vi "Log.vi"(7 "Enum Coordenadas":T4, 8 "Error In":errorcluster, 9 "Confirmação":bool, 10 "Log States":T5, 11 "DataIn":T1={"Quem Joga"="", "Tabuleiro"={"(0,0)"="", "(1,0)"="", "(0,1)"="", "(1,1)"="", "(2,0)"="", "(1,2)"="", "(2,2)"="", "(0,2)"="", "(2,1) "=""}, "GameOption"=enum."Multiplayer local", "Turno"=FALSE, "Player"="", "Player 1"="", "Player 2"="", "Dificuldade"=enum."Easy", "Table"=[], "Row"=0, "Aceitar Convite"=FALSE, "Inviter line"=0, "diretório"=path "", "Logout - panel close"=FALSE, "StartGame"=FALSE, "MatchData.lvclass"=refnum, "GameMode"=enum."Single Easy", "Level State"=FALSE}) -> (0 "Error Out":errorcluster, 3 "DataIn 2":T1={"Quem Joga"="", "Tabuleiro"={"(0,0)"="", "(1,0)"="", "(0,1)"="", "(1,1)"="", "(2,0)"="", "(1,2)"="", "(2,2)"="", "(0,2)"="", "(2,1) "=""}, "GameOption"=enum."Multiplayer local", "Turno"=FALSE, "Player"="", "Player 1"="", "Player 2"="", "Dificuldade"=enum."Easy", "Table"=[], "Row"=0, "Aceitar Convite"=FALSE, "Inviter line"=0, "diretório"=path "", "Logout - panel close"=FALSE, "StartGame"=FALSE, "MatchData.lvclass"=refnum, "GameMode"=enum."Single Easy", "Level State"=FALSE})   [LabVIEW 2018]
doc: "SubVI criada para fazer o log do histórico de partida jogada a jogada, registrando o vencedor."
uses:
  controls/LogStates.ctl
  controls/TabuleiroCoordenadas.ctl
  controls/DataIn.ctl
  MatchDataClasses/MatchData/MatchData.lvclass
  controls/Tabuleiro.ctl
  controls/Table.ctl
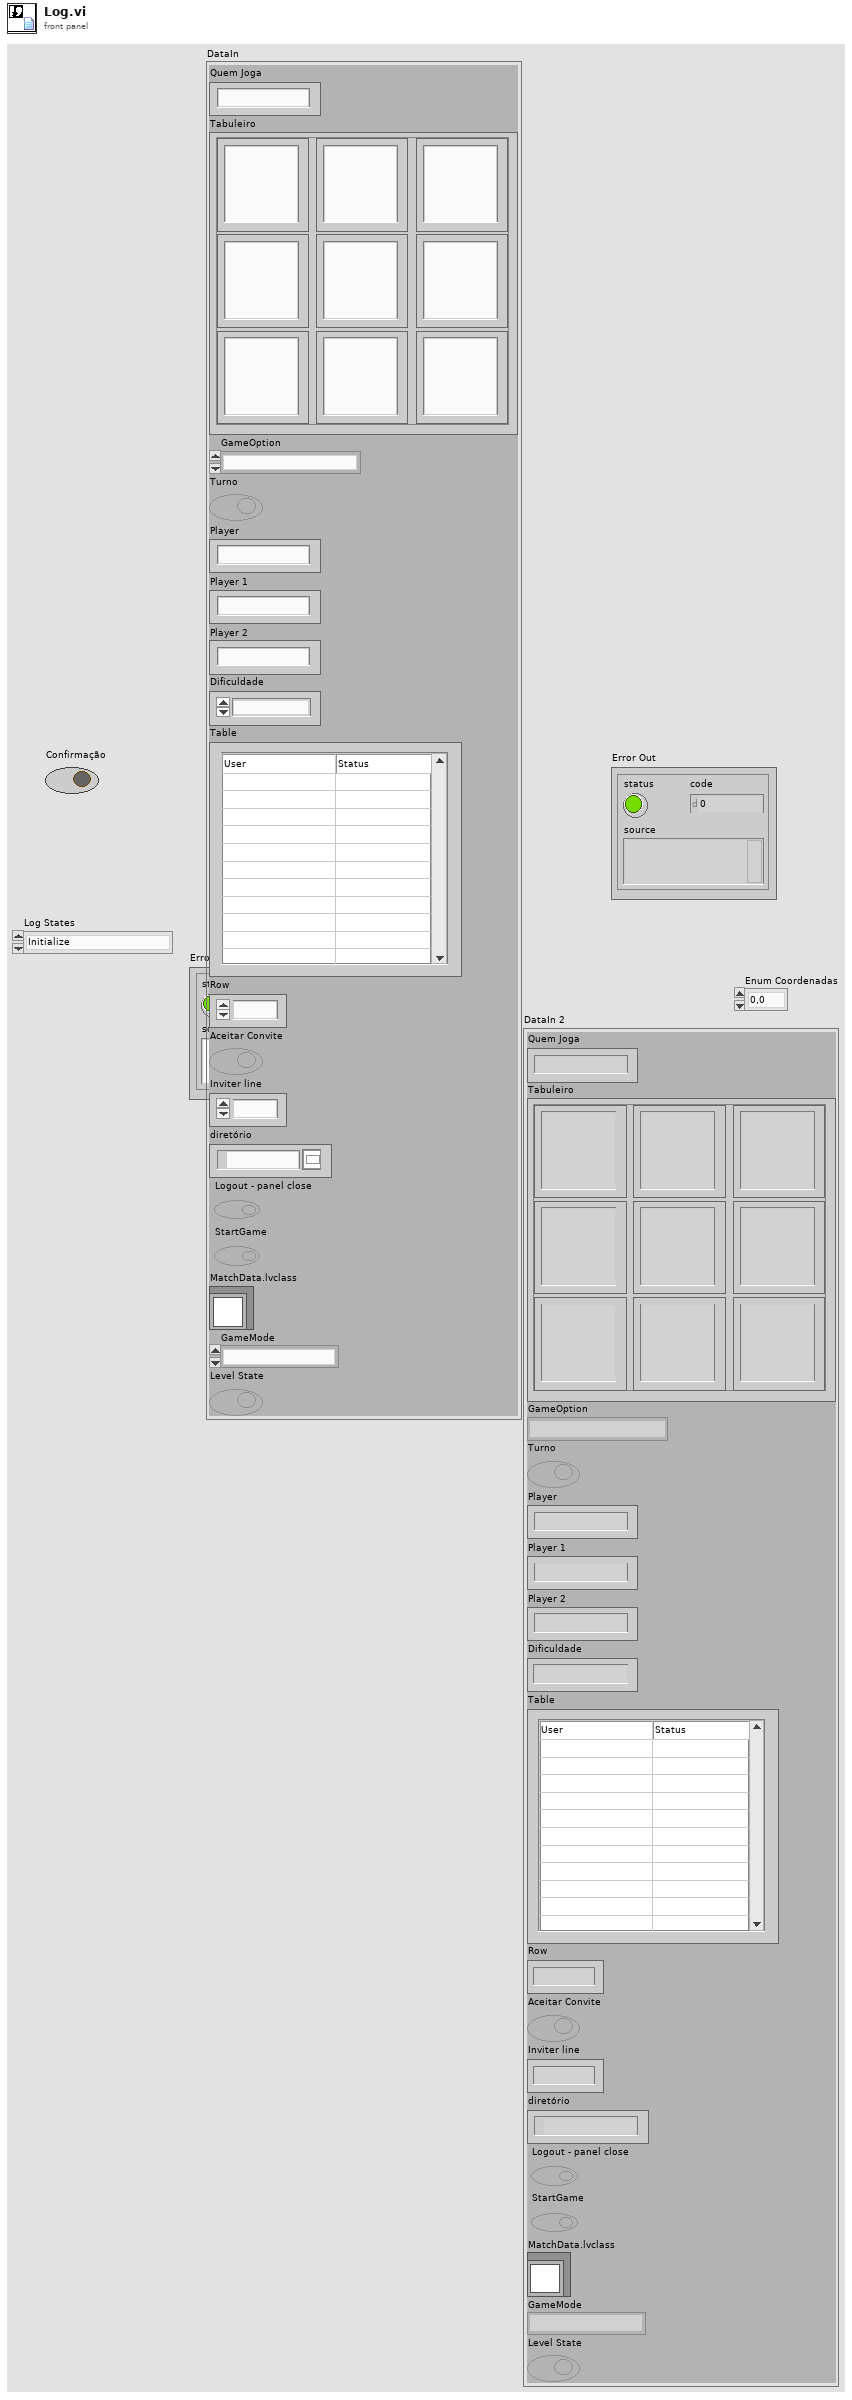
[diagram p1: front panel]
types:
  T1 = typedef "DataIn.ctl" = cluster{"Quem Joga":string, "Tabuleiro":T2, "GameOption":enum16{"Single Player", "Multiplayer local", "Multiplayer remoto", "Wait for Event", "Initialize", "Stop"}, "Turno":bool, "Player":string, "Player 1":string, "Player 2":string, "Dificuldade":enum16{"Easy", "Medium", "Hard"}, "Table":T3, "Row":u32, "Aceitar Convite":bool, "Inviter line":u32, "diretório":path, "Logout - panel close":bool, "StartGame":bool, "MatchData.lvclass":refnum<class "MatchData.lvclass">, "GameMode":enum16{"Single Easy", "Single Medium", "Single Hard", "Local", "Remote"}, "Level State":bool}
  T2 = typedef "Tabuleiro.ctl" = cluster{"(0,0)":string, "(1,0)":string, "(0,1)":string, "(1,1)":string, "(2,0)":string, "(1,2)":string, "(2,2)":string, "(0,2)":string, "(2,1) ":string}
  T3 = typedef "Table.ctl" = string[][]
  T4 = typedef "TabuleiroCoordenadas.ctl" = enum16{"0,0", "0,1", "0,2", "1,0", "1,1", "1,2", "2,0", "2,1", "2,2"}
  T5 = typedef "LogStates.ctl" = enum16{"Initialize", "Write", "Write (win, draw)", "Write (PC first)", "Write (Player first)", "Close"}
  T6 = enum16{"open", "replace", "create", "open or create", "replace or create", "replace or create with confirmation"}
  T7 = enum16{"Single Player", "Multiplayer local", "Multiplayer remoto", "Wait for Event", "Initialize", "Stop"}
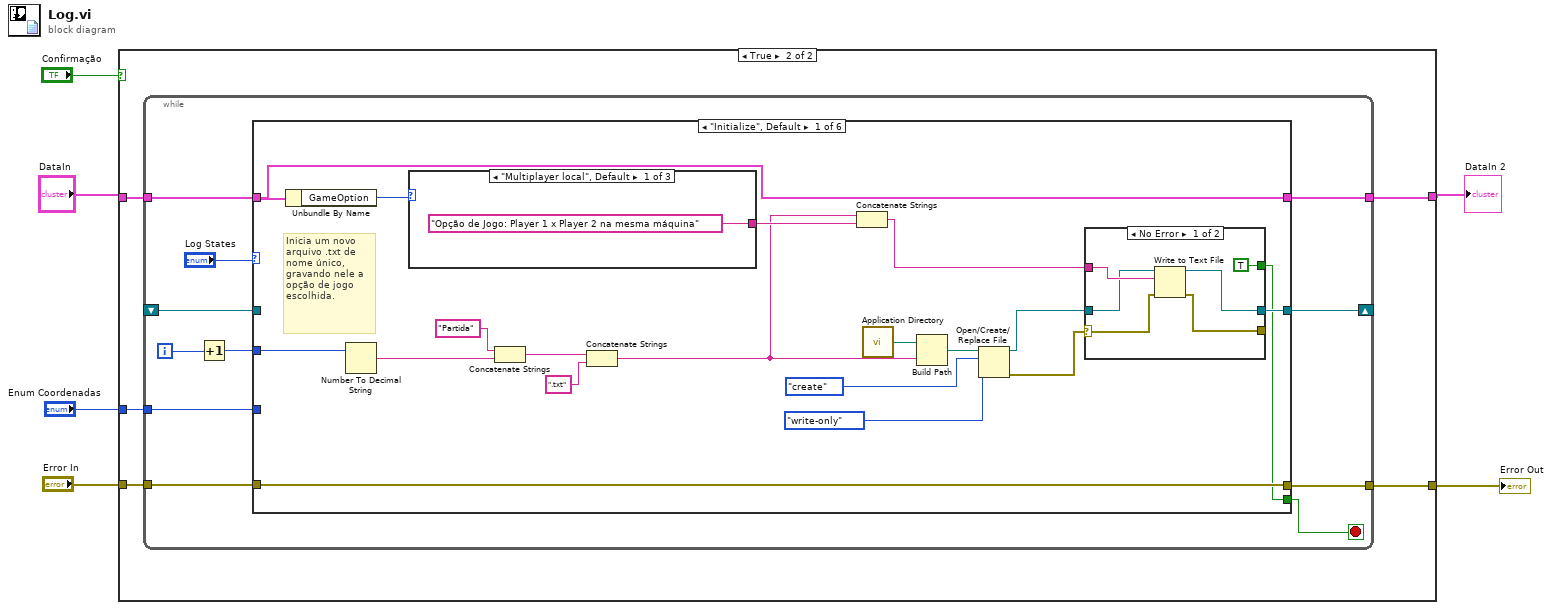
[diagram p0: block diagram]
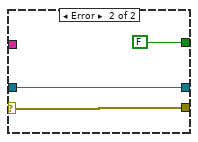
[diagram p3: hidden frame]
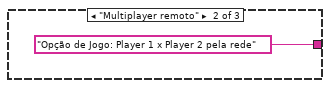
[diagram p4: hidden frame]
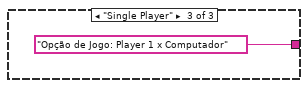
[diagram p5: hidden frame]
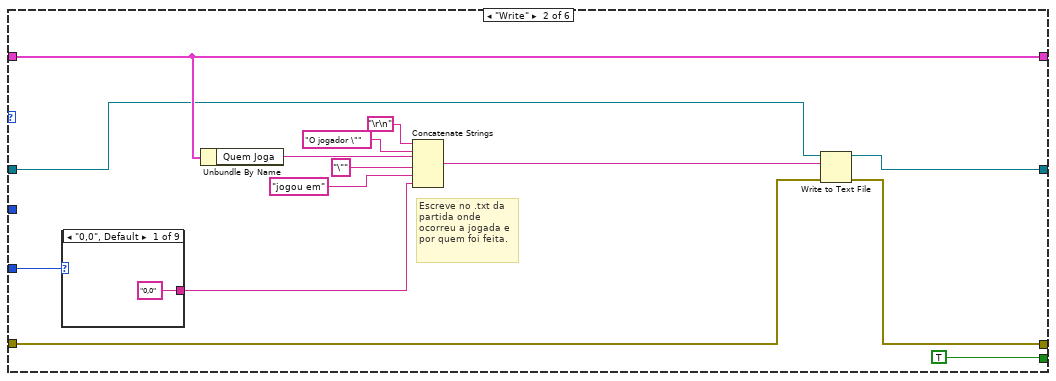
[diagram p6: hidden frame]
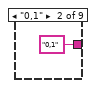
[diagram p7: hidden frame]
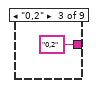
[diagram p8: hidden frame]
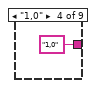
[diagram p9: hidden frame]
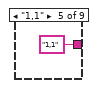
[diagram p10: hidden frame]
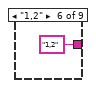
[diagram p11: hidden frame]
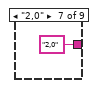
[diagram p12: hidden frame]
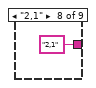
[diagram p13: hidden frame]
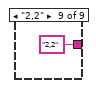
[diagram p14: hidden frame]
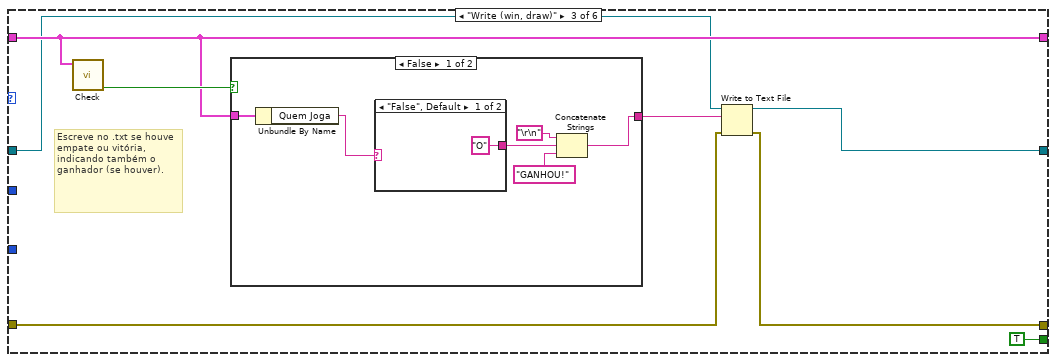
[diagram p15: hidden frame]
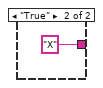
[diagram p16: hidden frame]
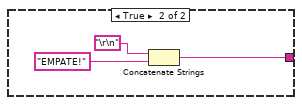
[diagram p17: hidden frame]
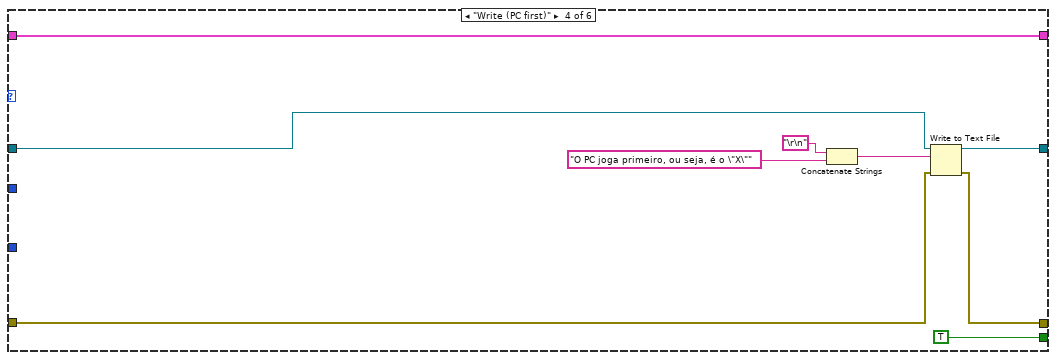
[diagram p18: hidden frame]
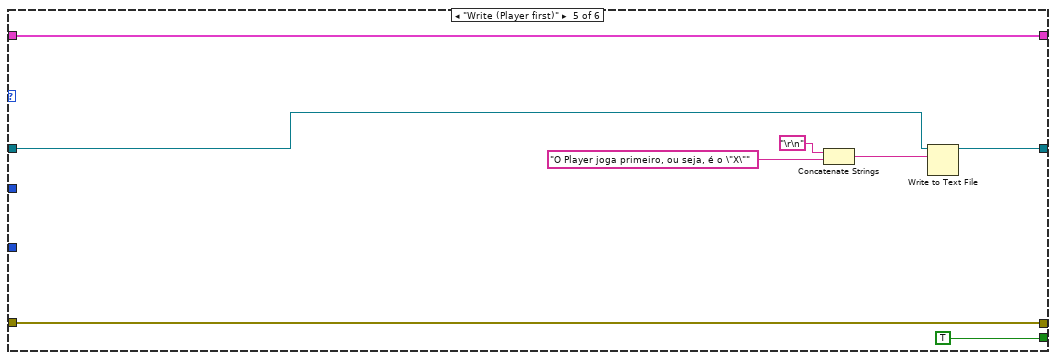
[diagram p19: hidden frame]
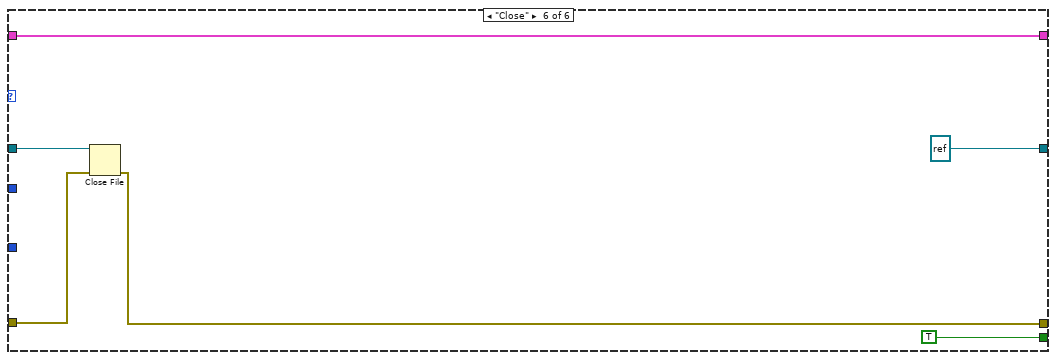
[diagram p20: hidden frame]
diagram:
  n1 = case shown="True" "Confirmação" {
    tunnel: "DataIn" -> [w8 w13]
    tunnel: "Error In" -> [w7 w12]
    tunnel: "Enum Coordenadas" -> [_ w11]
    tunnel: [w8 w10] -> w1
    tunnel: [w7 w9] -> w3
    frame False {
    }
    frame True {
      n2 = while {
        tunnel: w13 -> [w21]
        tunnel: w12 -> [w19]
        tunnel: w11 -> [w20]
        shift-right: [w18] -> _
        shift-left: _ -> [w17]
        tunnel: [w16] -> w10
        tunnel: [w15] -> w9
        i -> [w23]
        stop <- w14 stop-if-true
        n3 = Increment(x=w23) -> (x+1=w22:i32)
        n4 = case shown="\"Initialize\", Default" "Log States" {
          tunnel: w22 -> [w41 _ _ _ _ _]
          tunnel: w21 -> [w43 w65 w84 w106 w114 w117]
          tunnel: w20 -> [_ w68 _ _ _ _]
          tunnel: w19 -> [w26 w59 w82 w103 w113 w118]
          tunnel: [w27 w56 w80 w104 w108 refnum<file> refnum ("refnum out")] -> w18
          tunnel: w17 -> [_ w57 w79 w98 w107 w119]
          tunnel: [w43 w65 w84 w106 w114 w117] -> w16
          tunnel: [w26 w58 w81 w102 w113 w116] -> w15
          tunnel: [w25 TRUE TRUE TRUE TRUE TRUE] -> w14
          frame "Initialize", Default {
            # "Inicia um novo arquivo .txt de nome único, gravando nele a opção de jogo escolhida."
            n5 = Unbundle By Name(w43) -> ("GameOption"=w42:T7)
            n6 = Number To Decimal String(number=w41) -> (decimal integer string=w39:string)  [unwired: 1 in]
            n7 = case shown="\"Multiplayer local\", Default" w42 {
              tunnel: ["Opção de Jogo: Player 1 x Player 2 na mesma máquina" "Opção de Jogo: Player 1 x Player 2 pela rede" "Opção de Jogo: Player 1 x Computador"] -> w34
              frame "Multiplayer local", Default {
              }
              frame "Multiplayer remoto" {
              }
              frame "Single Player" {
              }
            }
            n8 = Concatenate Strings("Partida" ("string"), w39) -> (w38:string)
            n9 = Concatenate Strings(w38, ".txt" ("string")) -> (w33:string)
            n10 = Concatenate Strings(w33, w34) -> (w28:string)
            n11 = call <vilib>:"Application Directory.vi"() -> ("Application Directory"=w36:path)
            n12 = Build Path(base path=w36, name or relative path=w33) -> (appended path=w35:path)
            n13 = Open/Create/Replace File(file path (use dialog)=w35, operation (0:open)=T6."create", access (0:read/write)=enum16{"read/write", "read-only", "write-only"}."write-only") -> (refnum out=w29:refnum<file>, error out=w30:errorcluster)  [unwired: 3 in, 1 out]
            n14 = case shown="No Error" w30 {
              selector: w30 -> [w47 w50]
              tunnel: w29 -> [w48 w51]
              tunnel: w28 -> [w49 _]
              tunnel: [TRUE FALSE] -> w25
              tunnel: [w45 w51] -> w27
              tunnel: [w46 w50] -> _
              frame No Error {
                n15 = Write to Text File(file (use dialog)=w48, text=w49, error in=w47) -> (refnum out=w45:refnum<file>, error out=w46:errorcluster)  [unwired: 1 in, 1 out]
              }
              frame Error {
              }
            }
          }
          frame "Write" {
            # "Escreve no .txt da partida onde ocorreu a jogada e por quem foi feita."
            n16 = case shown="\"0,0\", Default" w68 {
              tunnel: ["0,0" "0,1" "0,2" "1,0" "1,1" "1,2" "2,0" "2,1" "2,2"] -> w61
              frame "0,0", Default {
              }
              frame "0,1" {
              }
              frame "0,2" {
              }
              frame "1,0" {
              }
              frame "1,1" {
              }
              frame "1,2" {
              }
              frame "2,0" {
              }
              frame "2,1" {
              }
              frame "2,2" {
              }
            }
            n17 = Unbundle By Name(w65) -> ("Quem Joga"=w64:string)
            n18 = Concatenate Strings("\r\n", "O jogador \"" ("string"), w64, "\"" ("string"), "jogou em" ("string"), w61) -> (w60:string)
            n19 = Write to Text File(file (use dialog)=w57, text=w60, error in=w59) -> (refnum out=w56:refnum<file>, error out=w58:errorcluster)  [unwired: 1 in, 1 out]
          }
          frame "Write (win, draw)" {
            # "Escreve no .txt se houve empate ou vitória, indicando também o ganhador (se houver)."
            n20 = call "Check.vi"("DataIn"=w84) -> ("True = Empatou"=w85:bool)  [unwired: 9 in, 1 out]
            n21 = case shown="False" w85 {
              tunnel: w84 -> [w92 _]
              tunnel: [w87 w95] -> w83
              frame False {
                n22 = Unbundle By Name(w92) -> ("Quem Joga"=w91:string)
                n23 = case shown="\"False\", Default" w91 {
                  tunnel: ["O" "X"] -> w90
                  frame "False", Default {
                  }
                  frame "True" {
                  }
                }
                n24 = Concatenate Strings("\r\n", w90, "GANHOU!" ("string")) -> (w87:string)
              }
              frame True {
                n25 = Concatenate Strings("\r\n", "EMPATE!" ("string")) -> (w95:string)
              }
            }
            n26 = Write to Text File(file (use dialog)=w79, text=w83, error in=w82) -> (refnum out=w80:refnum<file>, error out=w81:errorcluster)  [unwired: 1 in, 1 out]
          }
          frame "Write (PC first)" {
            n27 = Concatenate Strings("\r\n", "O PC joga primeiro, ou seja, é o \"X\"" ("string")) -> (w101:string)
            n28 = Write to Text File(file (use dialog)=w98, text=w101, error in=w103) -> (refnum out=w104:refnum<file>, error out=w102:errorcluster)  [unwired: 1 in, 1 out]
          }
          frame "Write (Player first)" {
            n29 = Concatenate Strings("\r\n", "O Player joga primeiro, ou seja, é o \"X\"" ("string")) -> (w111:string)
            n30 = Write to Text File(file (use dialog)=w107, text=w111) -> (refnum out=w108:refnum<file>)  [unwired: 2 in, 2 out]
          }
          frame "Close" {
            n31 = Close File(refnum=w119, error in=w118) -> (error out=w116:errorcluster)  [unwired: 1 out]
          }
        }
      }
    }
  }
  "Error Out" <- w3
  "DataIn 2" <- w1
